vi "Cleanup Stack.vi"(8 "error in (no error)":errorcluster, 11 "IP Connection in":refnum<class "IP Connection.lvclass">) -> (0 "error out":errorcluster, 3 "IP Connection out":refnum<class "IP Connection.lvclass">)   [LabVIEW 2011, in "Tinkerforge.lvlib" / "IP Connection.lvclass"]
doc: "This VI removes all devices from the stack and releases all synchronization objects of the devices in stack."
uses:
  IP Connection.lvclass
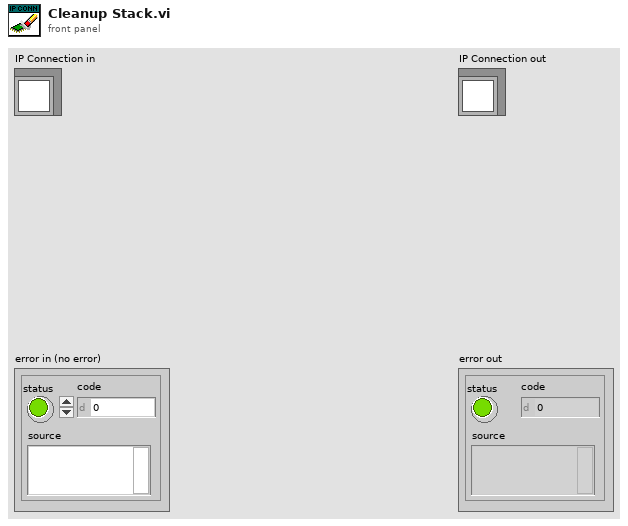
[diagram p1: front panel]
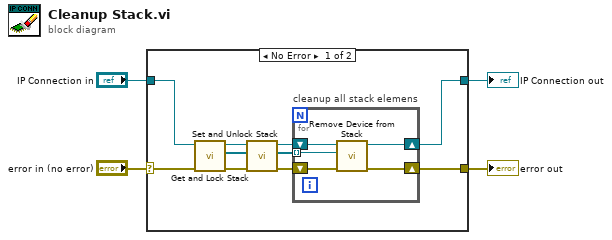
[diagram p0: block diagram]
diagram:
  n1 = case shown="No Error" "error in (no error)" {
    selector: "error in (no error)" -> [w13 w20]
    tunnel: [w12 w20] -> w3
    tunnel: [w5 w19] -> w1
    tunnel: "IP Connection in" -> [w6 w19]
    frame No Error {
      n2 = call "Get and Lock Stack.vi"("error in (no error)"=w13, "IP Connection in"=w6) -> ("error out"=w11:errorcluster, "Stack"=w10:refnum<class "Device.lvclass">[], "IP Connection out"=w9:refnum<class "IP Connection.lvclass">)  [unwired: 7 in]
      n3 = call "Set and Unlock Stack.vi"("error in (no error)"=w11, "Stack"=w10, "IP Connection in"=w9) -> ("error out"=w7:errorcluster, "IP Connection out"=w8:refnum<class "IP Connection.lvclass">)  [unwired: 7 in]
      n4 = for "cleanup all stack elemens" {
        tunnel: w10 -> [w17] mode=indexing
        shift-right: [w14] -> w12
        shift-left: w7 -> [w18]
        shift-right: [w15] -> w5
        shift-left: w8 -> [w16]
        n5 = call "Remove Device from Stack.vi"("error in (no error)"=w18, "Device in"=w17, "IP Connection in"=w16) -> ("error out"=w14:errorcluster, "IP Connection out"=w15:refnum<class "IP Connection.lvclass">)  [unwired: 7 in]
      }
    }
    frame Error {
    }
  }
  "error out" <- w3
  "IP Connection out" <- w1
